vi "Handle Error.vi"(8 "error in (no error)":errorcluster, 11 "Test Executive Builder in":refnum<class "Test Executive Builder.lvclass">) -> (0 "error out":errorcluster, 2 "stop actor?":bool=TRUE, 3 "Test Executive Builder out":refnum<class "Test Executive Builder.lvclass">)   [LabVIEW 2019, in "Test Executive Builder.lvclass"]
doc: "(<B>Filename</B>: Actor Framework.lvlib:Actor.lvclass:Handle Error.vi)\n\nDefines how the actor handles an error that occurred while processing a message. By default, this method does nothing except stop the actor."
uses:
  <vilib>/gpm_packages/@cs/Test-executive-builder/Example/Application/Test Executive Builder/Test Executive Builder/Test Executive Builder.lvclass
  <vilib>/gpm_packages/@cs/Test-executive-builder/Source/Test Executive Builder Model/Test Executive Builder Model/Test Executive Builder Model.lvclass
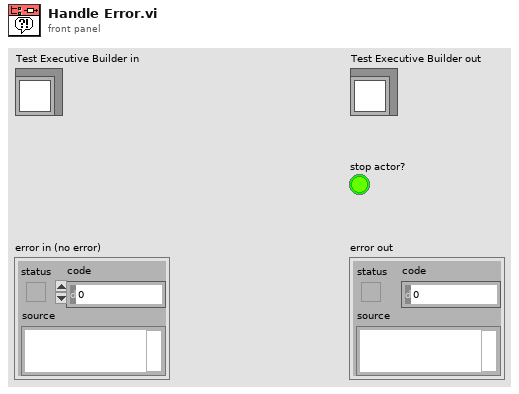
[diagram p1: front panel]
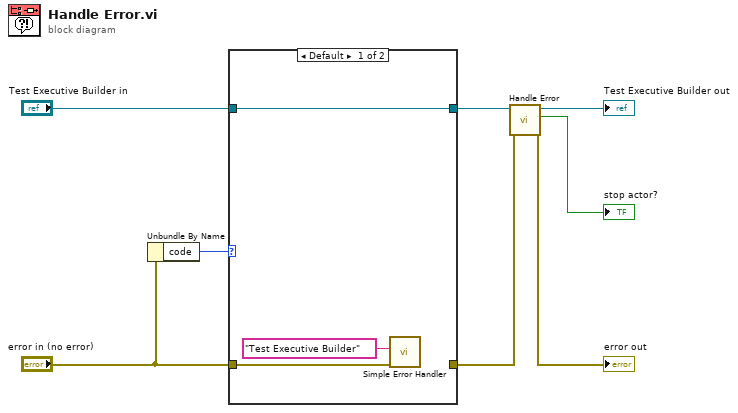
[diagram p0: block diagram]
diagram:
  n1 = Unbundle By Name("error in (no error)") -> ("code"=w6:i32)
  n2 = case shown="Default" w6 {
    tunnel: [w11 w13] -> w4
    tunnel: "Test Executive Builder in" -> [w11 w13]
    tunnel: "error in (no error)" -> [w10 w12]
    tunnel: [_ w12] -> w2
    frame Default {
      n3 = call <vilib>:"Simple Error Handler.vi"("error source (\" \")"="Test Executive Builder" ("error source (\" \")"), "error in (no error)"=w10) -> ()  [unwired: 3 in, 5 out]
    }
    frame 43, 1608 {
    }
  }
  n4 = call-parent "Handle Error.vi"("error in (no error)"=w2, "IModel in"=w4) -> ("error out"=→"error out":errorcluster, "stop actor?"=→"stop actor?":bool, "IModel out"=→"Test Executive Builder out":refnum<class "Test Executive Builder.lvclass">)  [unwired: 7 in]
